vi "LOER_GetAutoToolRegions.vi"(0 "XRef":T9, 1 "State In":T7={"Inputs"=1, "SelectedIndex"=0, "ClassInfo"=[], "Width"=100, "EventReg Type"=variant}) -> (14 "Regions":T2, 15 "Fatal Error Out":T1)   [LabVIEW 2016, in "LV Object Event Registration Node.xnode"]
uses:
  LV Object Event Registration Node.xnode
  <vilib>/XNodeSupport/XNodeXNodeRef.ctl
  LOER_State.ctl
  LOER_ClassInfo.ctl
  <vilib>/XNodeSupport/XNodeAutotoolRegions.ctl
  <vilib>/XNodeSupport/XNodeAutotoolRegion.ctl
  <vilib>/XNodeSupport/XNodeRect32.ctl
  <vilib>/XNodeSupport/XNodeInt.ctl
  <vilib>/XNodeSupport/XNodeTools.ctl
  <vilib>/XNodeSupport/XNodeErrorCluster.ctl
  <vilib>/XNodeSupport/NI_XNodeSupport.lvlib
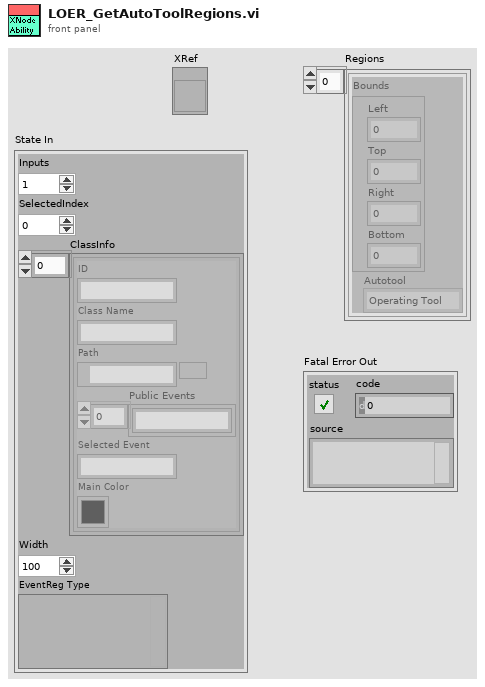
[diagram p1: front panel]
types:
  T1 = typedef "NI_XNodeSupport.lvlib/XNodeErrorCluster.ctl" = errorcluster
  T2 = typedef "NI_XNodeSupport.lvlib/XNodeAutotoolRegions.ctl" = T3[]
  T3 = typedef "NI_XNodeSupport.lvlib/XNodeAutotoolRegion.ctl" = cluster{"Bounds":T4, "Autotool":T6}
  T4 = typedef "NI_XNodeSupport.lvlib/XNodeRect32.ctl" = cluster{"Left":T5, "Top":T5, "Right":T5, "Bottom":T5}
  T5 = typedef "NI_XNodeSupport.lvlib/XNodeInt.ctl" = i32
  T6 = typedef "NI_XNodeSupport.lvlib/XNodeTools.ctl" = enum32{"Operating Tool", "Placement Tool", "Labelling Tool", "Wiring Tool", "Scroll Tool", "Breakpoint Tool", "Probe Tool", "Auto Tool"}
  T7 = typedef "LV Object Event Registration Node.xnode/LOER_State.ctl" = cluster{"Inputs":u16, "SelectedIndex":i16, "ClassInfo":T8[], "Width":u16, "EventReg Type":variant}
  T8 = typedef "LV Object Event Registration Node.xnode/LOER_ClassInfo.ctl" = cluster{"ID":string, "Class Name":string, "Path":path, "Public Events":string[], "Selected Event":string, "Main Color":u32}
  T9 = typedef "NI_XNodeSupport.lvlib/XNodeXNodeRef.ctl" = refnum<vi>
  T10 = typedef "NI_XNodeSupport.lvlib/XNodeBounds.ctl" = cluster{"Width":T5, "Height":T5}
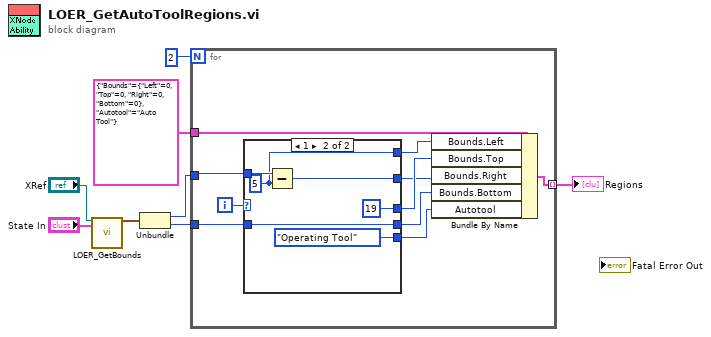
[diagram p0: block diagram]
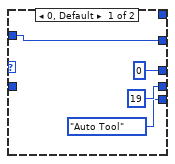
[diagram p2: hidden frame]
diagram:
  n1 = call "LOER_GetBounds.vi"("XRef"="XRef", "State In"="State In") -> ("Bounds"=w6:T10)  [unwired: 16 in, 1 out]
  n2 = Unbundle(w6) -> ("Width"=w3:T5, "Height"=w2:T5)
  n3 = for {
    N: 2 -> [_]
    tunnel: T3 {"Bounds"={"Left"=0, "Top"=0, "Right"=0, "Bottom"=0}, "Autotool"=enum."Auto Tool"} ("Autotool Region") -> [w18]
    tunnel: w3 -> [w11]
    tunnel: w2 -> [w13]
    tunnel: [w12] -> w1 mode=indexing
    i -> [w17]
    n4 = case shown="1" w17 {
      tunnel: [0 19] -> w16
      tunnel: [19 w26] -> w15
      tunnel: [XNodeTools."Auto Tool" ("Autotool") XNodeTools."Operating Tool" ("Autotool")] -> w14
      tunnel: w13 -> [_ w26]
      tunnel: w11 -> [w19 w25]
      tunnel: [w19 w24] -> w10
      tunnel: [_ w23] -> w9
      frame 0, Default {
      }
      frame 1 {
        w23 = T5 5 ("y")
        n5 = Subtract(x=w25, y=w23) -> (x-y=w24:T5)
      }
    }
    n6 = Bundle By Name(cluster=w18, "Bounds.Left"=w9, "Bounds.Top"=w16, "Bounds.Right"=w10, "Bounds.Bottom"=w15, "Autotool"=w14) -> (w12:T3)
  }
  "Regions" <- w1
